vi "main.vi"() -> ()   [LabVIEW 2019]
uses:
  Controls/Estats.ctl
panel:
  out "Numeric":i32
  in  "stop":bool
  out "Boolean":bool
  # "fixar-se en l'execució és molt lenta, veure el main elapsed loop"
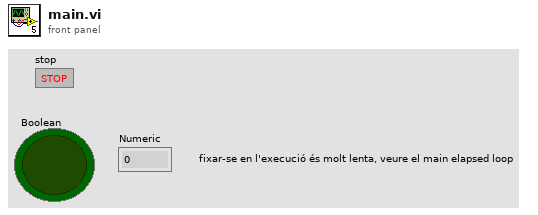
[diagram p1: front panel]
types:
  T1 = typedef "Estats.ctl" = enum16{"inicialitza", "Estat1", "Estat2"}
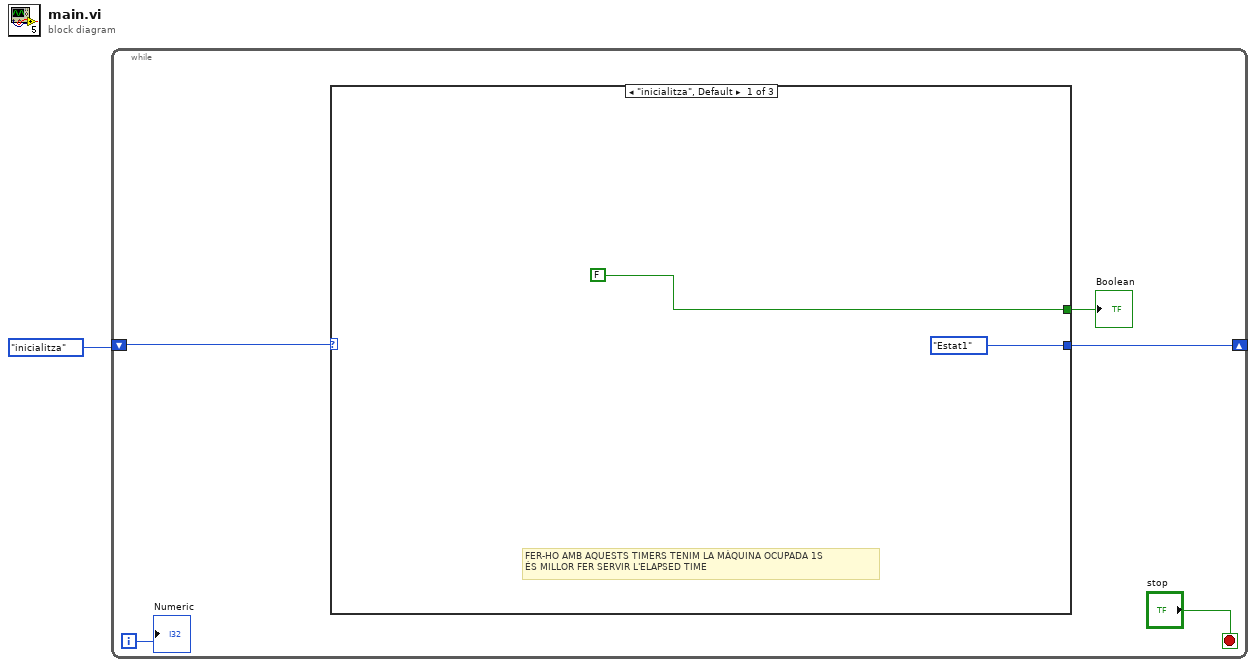
[diagram p0: block diagram]
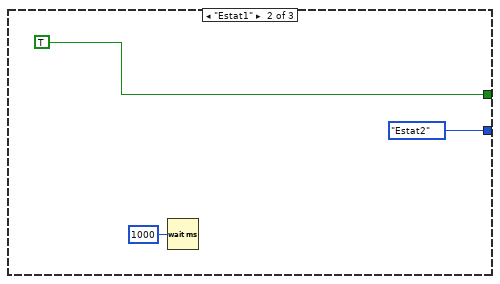
[diagram p2: hidden frame]
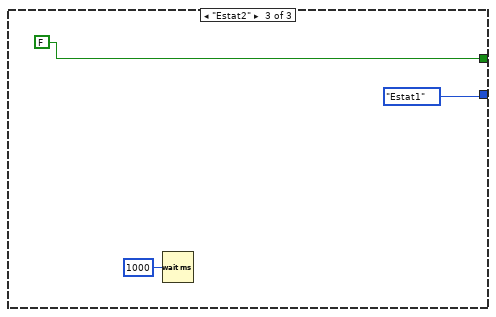
[diagram p3: hidden frame]
diagram:
  n1 = while {
    shift-right: [w5] -> _
    shift-left: Estats."inicialitza" ("Enum") -> [w6]
    i -> [w2]
    stop <- "stop" stop-if-true
    n2 = case shown="\"inicialitza\", Default" w6 {
      tunnel: [Estats."Estat1" ("Enum") Estats."Estat2" ("Enum") Estats."Estat1" ("Enum")] -> w5
      tunnel: [FALSE ("Boolean") TRUE ("Boolean") FALSE ("Boolean")] -> w3
      frame "inicialitza", Default {
        # "FER-HO AMB AQUESTS TIMERS TENIM LA MÀQUINA OCUPADA 1S\nÉS MILLOR FER SERVIR L'ELAPSED TIME"
      }
      frame "Estat1" {
        n3 = Wait (ms)(milliseconds to wait=u32 1000) -> ()  [unwired: 1 out]
      }
      frame "Estat2" {
        n4 = Wait (ms)(milliseconds to wait=u32 1000) -> ()  [unwired: 1 out]
      }
    }
    "Boolean" <- w3
    "Numeric" <- w2
  }
